vi "FAS.vi"() -> ()   [LabVIEW 2019]
uses:
  <vilib>/MakerHub/LINX/Public/Peripherals/Digital/Digital Read 1 Chan.vi
  <vilib>/MakerHub/LINX/Public/Peripherals/Digital/Digital Write 1 Chan.vi
  <vilib>/MakerHub/LINX/Public/Peripherals/Digital/Digital Read N Chans.vi
  <vilib>/MakerHub/LINX/Public/Peripherals/Digital/Digital Write N Chans.vi
  <vilib>/MakerHub/LINX/Private/Local IO/LinxDigitalRead.vi
  <vilib>/MakerHub/LINX/Public/Utilities/Check Channel.vi
  <vilib>/MakerHub/LINX/Private/Local IO/LinxDigitalWrite.vi
  <vilib>/MakerHub/LINX/Public/Utilities/Open Serial.vi
  <vilib>/MakerHub/LINX/Private/Utilties/Generate Error.vi
  <vilib>/MakerHub/LINX/LMH-LINX.lvlib
panel:
  in  "Stop":bool
  in  "Serial Port":refnum<visa-resource-name>="N/A"
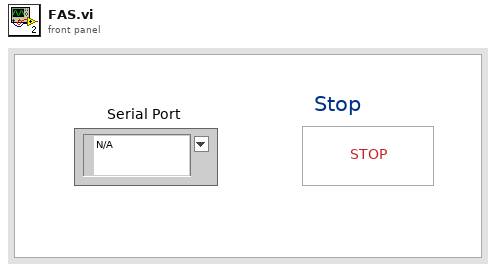
[diagram p1: front panel]
types:
  T1 = typedef "LMH-LINX.lvlib/LINX Ref.ctl" = cluster{"IO":T2, "Interface":T3, "LINX Device Config":T4}
  T2 = typedef "LMH-LINX.lvlib/Platform.ctl" = enum16{"Remote", "Local"}
  T3 = typedef "LMH-LINX.lvlib/Interface.ctl" = enum16{"Serial", "TCP"}
  T4 = typedef "LMH-LINX.lvlib/Device.lvlib/LINX Device Config.ctl" = cluster{"Interface":T3, "COM Port":refnum<visa-resource-name>, "TCP Configuration":T5, "Device Family":u8, "Device ID":u8, "Device Name":string, "TCP Ref":refnum<k5>, "Channels":T6}
  T5 = typedef "LMH-LINX.lvlib/Device.lvlib/TCP Config.ctl" = cluster{"IP Address":string, "Port":u16}
  T6 = typedef "LMH-LINX.lvlib/Channels.ctl" = cluster{"DI":u8[], "DO":u8[], "AI":u8[], "AO":u8[], "PWM":u8[], "QE":u8[], "UART":u8[], "I2C 2":u8[], "SPI":u8[], "CAN":u8[], "Servo":u8[], "AI Ref (V)":dbl, "AI Resolution (Bits)":u8, "AO Ref (V)":dbl, "AO Resolution (Bits)":u8}
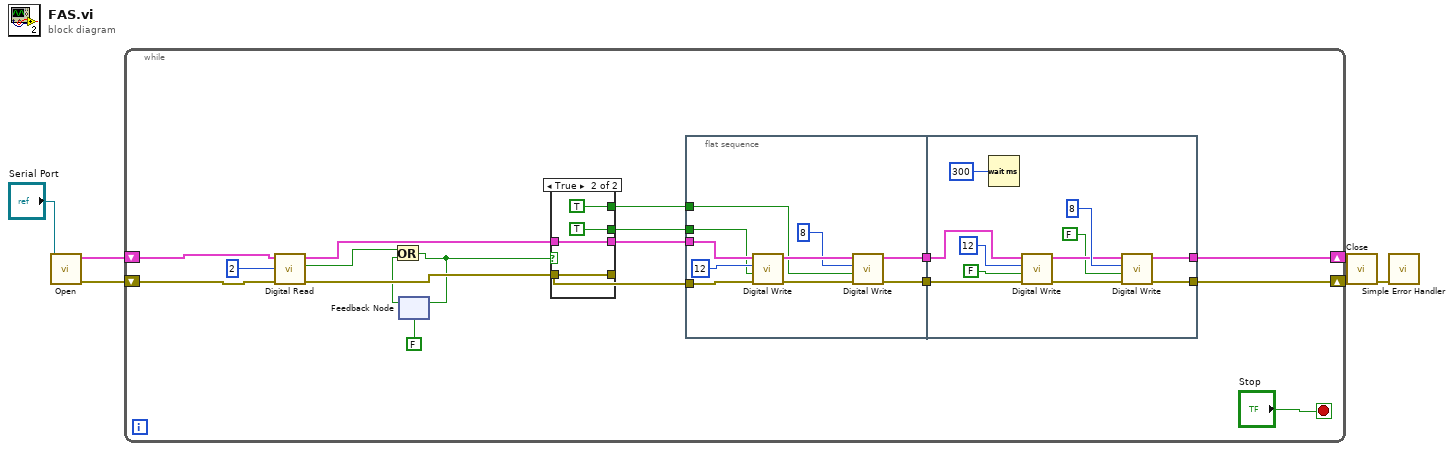
[diagram p0: block diagram]
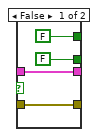
[diagram p2: hidden frame]
diagram:
  n1 = call-poly <vilib>:"Open.vi"("Serial Port"="Serial Port") -> ("Error Out"=w3:errorcluster, "LINX Resource"=w5:T1)  [unwired: 8 in, 1 out]
  n2 = while {
    shift-right: [w9] -> w2
    shift-left: w5 -> [w11]
    shift-right: [w8] -> w4
    shift-left: w3 -> [w10]
    stop <- "Stop" stop-if-true
    n3 = call-poly <vilib>:"Digital Read.vi"("Error In"=w10, "DI Channel"=u8 2, "LINX Resource"=w11) -> ("Error Out"=w23:errorcluster, "DI Value"=w15:bool, "LINX Resource"=w22:T1)  [unwired: 6 in]
    n4 = feedback #1(FALSE) -> (w13:bool)
    n5 = Or(x=w15, y=w13) -> (x .or. y?=w14:bool)
    n6 = feedback-in #1(w14) -> ()
    n7 = case shown="True" w14 {
      tunnel: [w48 w53] -> w18
      tunnel: w23 -> [w48 w53]
      tunnel: [w49 w52] -> w19
      tunnel: w22 -> [w49 w52]
      tunnel: [FALSE TRUE] -> w17
      tunnel: [FALSE TRUE] -> w16
      frame False {
      }
      frame True {
      }
    }
    n8 = flat-sequence {
      tunnel: [w33] -> w21
      tunnel: [w29] -> w20
      tunnel: w19 -> [w28]
      tunnel: w18 -> [w27]
      tunnel: w17 -> [w26]
      tunnel: w16 -> [w25]
      tunnel: w21 -> [w41]
      tunnel: w20 -> [w40]
      tunnel: [w36] -> w9
      tunnel: [w35] -> w8
      frame #0 {
        n9 = call-poly <vilib>:"Digital Write.vi"("Error In"=w27, "Output Value"=w26, "DO Channel"=u8 12, "LINX Resource"=w28) -> ("Error Out"=w32:errorcluster, "LINX Resource"=w34:T1)  [unwired: 6 in]
        n10 = call-poly <vilib>:"Digital Write.vi"("Error In"=w32, "Output Value"=w25, "DO Channel"=u8 8, "LINX Resource"=w34) -> ("Error Out"=w29:errorcluster, "LINX Resource"=w33:T1)  [unwired: 6 in]
      }
      frame #1 {
        n11 = Wait (ms)(milliseconds to wait=u32 300) -> ()  [unwired: 1 out]
        n12 = call-poly <vilib>:"Digital Write.vi"("Error In"=w40, "Output Value"=FALSE, "DO Channel"=u8 12, "LINX Resource"=w41) -> ("Error Out"=w43:errorcluster, "LINX Resource"=w42:T1)  [unwired: 6 in]
        n13 = call-poly <vilib>:"Digital Write.vi"("Error In"=w43, "Output Value"=FALSE, "DO Channel"=u8 8, "LINX Resource"=w42) -> ("Error Out"=w35:errorcluster, "LINX Resource"=w36:T1)  [unwired: 6 in]
      }
    }
  }
  n14 = call <vilib>:"Close.vi"("Error In"=w4, "LINX Resource"=w2) -> ("Error Out"=w6:errorcluster)  [unwired: 9 in]
  n15 = call <vilib>:"Simple Error Handler.vi"("error in (no error)"=w6) -> ()  [unwired: 4 in, 5 out]
